vi "Init.vi"(8 "error in (no error)":errorcluster, 11 "RHS_2D_VIRef":refnum<class "NI_RHS_2D_VIRef.lvclass">) -> (0 "error out":errorcluster, 3 "initialized RHS_2D_VIRef":refnum<class "NI_RHS_2D_VIRef.lvclass">)   [LabVIEW 2020, in "NI_PDE.lvlib" / "NI_RHS_2D_VIRef.lvclass"]
uses:
  <vilib>/gmath/pde.llb/RHSClass/RHS_2D_VIRef/NI_RHS_2D_VIRef.lvclass
  <vilib>/gmath/pde.llb/RHSClass/Class Type.ctl
  <vilib>/gmath/pde.llb/RHSClass/RHS_2D_VIRef/NI_RHS_2D_VIRef.lvclass/NI_RHS_2D_VIRef.ctl
  <vilib>/gmath/pde.llb/RHSClass/NI_RHS.lvclass
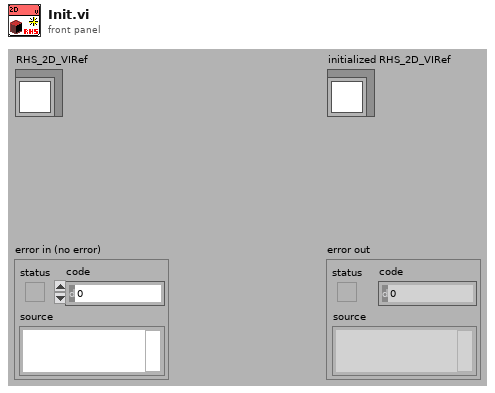
[diagram p1: front panel]
types:
  T1 = typedef "NI_PDE.lvlib/NI_RHS.lvclass/Class Type.ctl" = i32
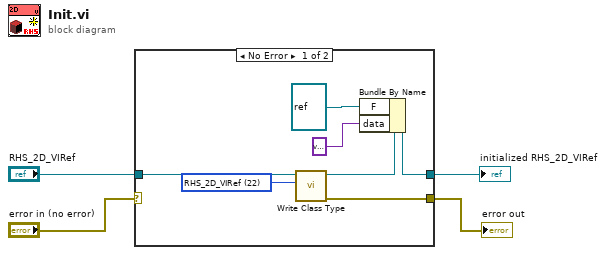
[diagram p0: block diagram]
diagram:
  n1 = case shown="No Error" "error in (no error)" {
    selector: "error in (no error)" -> [_ w13]
    tunnel: [w8 w12] -> w4
    tunnel: [w7 w13] -> w3
    tunnel: "RHS_2D_VIRef" -> [w10 w12]
    frame No Error {
      w11 = T1 22 items=["RHS"=0, "RHS_2D"=20, "RHS_2D_Numeric"=21, "RHS_2D_VIRef"=22, "RHS_3D"=30, "RHS_3D_Numeric"=31, "RHS_3D_VIRef"=32] ("RHS class type")
      n2 = call-dynamic "Write Class Type.vi"("RHS class type"=w11, "RHS.lvclass in"=w10) -> ("error out"=w7:errorcluster, "RHS.lvclass out"=w9:refnum<class "NI_RHS_2D_VIRef.lvclass">)  [unwired: 1 in, 7 out]
      n3 = Bundle By Name(cluster=w9, "F"=refnum<vi> refnum, "data"=variant) -> (w8:refnum<class "NI_RHS_2D_VIRef.lvclass">)
    }
    frame Error {
    }
  }
  "initialized RHS_2D_VIRef" <- w4
  "error out" <- w3
